vi "send&receive_2_arrs, call foo.vi"() -> ()   [LabVIEW 2018, in "LV2Julia_core.lvlib"]
uses:
  LV2Julia_core.lvlib
  Commands.ctl
  commands LV2Jl.ctl
  Server or client state.ctl
  d2cb43a9-9305-42fb-ad58-bce983510195.vi
  5398bb44-7854-4704-a5a4-70900ab1788b.vi
  4837e4b1-53a7-49b6-9aef-263877b89a45.vi
  464ea3ce-3b02-4d89-9aac-48d52021810b.vi
  edf81fa3-46bf-427f-9605-85b461656974.vi
  StackFrame.ctl
  detailed error info.ctl
panel:
  out "resp1":dbl
  in  "arg2":string
  in  "arg1":dbl
  in  "1D Array of I16":i16[](array[numeric])=[13, 7, 546]
  in  "2D Array of Cx32":csg[][](array[numeric])=[[3.0+0.0i, 1.0+1.0i], [0.0+7.0i, 1.0+4.0i]] format="%#_13g"
  out "resp2":i32[](array[numeric])
  in  "next":bool
  in  "stop LV only":bool
  in  "stop":bool
  out "detailed error info":T1
  out "resp3":dbl[](array[numeric])
  out "Jl Server state out":T3
  out "short err code":u8
  out "final error":errorcluster
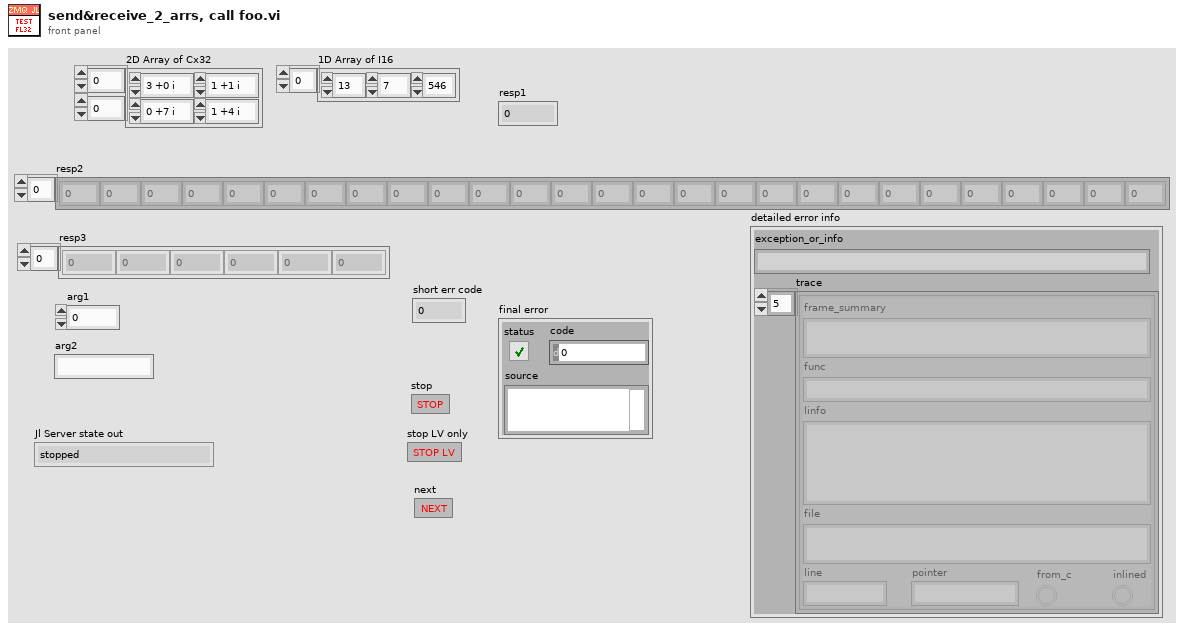
[diagram p1: front panel]
types:
  T1 = typedef "LV-0mq-Julia_roundtrip-lib.lvlib/detailed error info.ctl" = cluster{"exception_or_info":string, "trace":T2[]}
  T2 = typedef "LV-0mq-Julia_roundtrip-lib.lvlib/StackFrame.ctl" = cluster{"frame_summary":string, "func":string, "linfo":string, "file":string, "line":i32, "pointer":u64, "from_c":bool, "inlined":bool}
  T3 = typedef "LV-0mq-Julia_roundtrip-lib.lvlib/Server or client state.ctl" = enum16{"stopped", "running", "unknown"}
  T4 = typedef "LV-0mq-Julia_roundtrip-lib.lvlib/Commands.ctl" = enum16{"Start Jl-server & Init LV-client", "Send request & Get response ", "Stop Jl-server & Cleanup LV-client", "Cleanup LV-client", "Start Jl-server", "Stop Jl-server", "Init LV-Client", "Cleanup LV-Client", "(not allowed)", "Set LV Client state", "Set Jl Server state", "set ZMQ timeout", "read ZMQ timeout", "read-out state"}
  T5 = typedef "LV-0mq-Julia_roundtrip-lib.lvlib/commands LV2Jl.ctl" = u8
  T6 = typedef "LV-0mq-Julia_roundtrip-lib.lvlib/Bindata&description.ctl" = cluster{"bindata_descr":T7[], "bindata":u8[]}
  T7 = typedef "LV-0mq-Julia_roundtrip-lib.lvlib/Bindata description.ctl" = cluster{"nofbytes":i32, "numtype":string, "start":i32, "arrdims":i32[], "kwarg_name":string, "category":string}
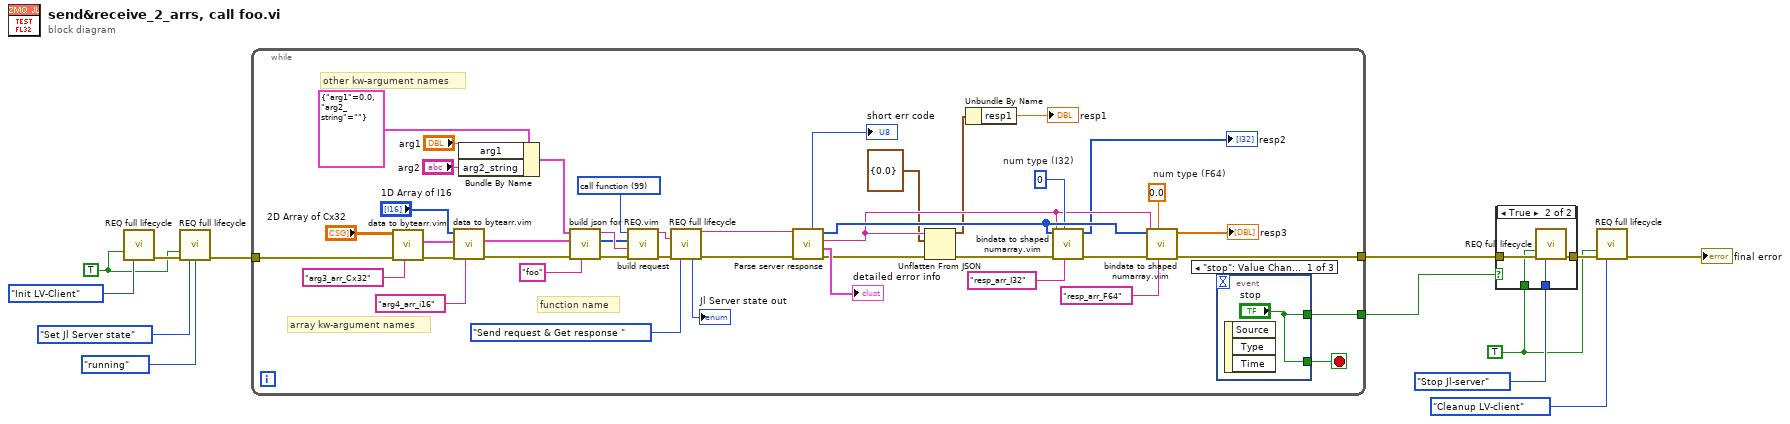
[diagram p0: block diagram]
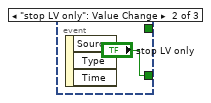
[diagram p2: hidden frame]
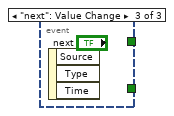
[diagram p3: hidden frame]
diagram:
  w4 = TRUE ("Force command")
  w8 = TRUE ("Force command")
  n1 = call "REQ full lifecycle.vi"("Force command"=w4, "command"=Commands."Init LV-Client") -> ("error out"=w6:errorcluster)  [unwired: 7 in, 6 out]
  n2 = call "REQ full lifecycle.vi"("Force command"=w4, "error in"=w6, "command"=Commands."Set Jl Server state", "Jl Server state in"=Server_or_client_state."running") -> ("error out"=w2:errorcluster)  [unwired: 5 in, 6 out]
  n3 = while {
    tunnel: w2 -> [w25]
    tunnel: [w41] -> w13
    tunnel: [w42] -> w1
    stop <- w43 stop-if-true
    w37 = 0  # num type (I32)
    w40 = 0.0  # num type (F64)
    w50 = T5 99 items=["call function"=99, "ping"=112, "stop"=115] ("Command")
    # "function name"
    # "other kw-argument names"
    # "array kw-argument names"
    n4 = call "data to bytearr.vim"("kwarg_name"="arg3_arr_Cx32", "error in (no error)"=w25, "data in"="2D Array of Cx32") -> ("error out"=w29:errorcluster, "Bindata & descr out"=w28:T6)  [unwired: 6 in, 1 out]
    n5 = call "data to bytearr.vim"("kwarg_name"="arg4_arr_i16", "error in (no error)"=w29, "Bindata & descr in"=w28, "data in"="1D Array of I16") -> ("error out"=w26:errorcluster, "Bindata & descr out"=w27:T6)  [unwired: 5 in, 1 out]
    n6 = Bundle By Name(cluster=cluster{"arg1":dbl, "arg2_string":string} {"arg1"=0.0, "arg2_string"=""}, "arg1"="arg1", "arg2_string"="arg2") -> (w21:cluster{"arg1":dbl, "arg2_string":string})
    n7 = call "build json for REQ.vim"("fun2call"="foo", "Bindata & descr in"=w27, "error in (no error)"=w26, "Arguments 1"=w21) -> ("error out"=w55:errorcluster, "bindata out"=w46:u8[], "JSON string out"=w47:string)  [unwired: 5 in]
    n8 = call "build request.vi"("error in (no error)"=w55, "JSON data"=w47, "binary data"=w46, "Command"=w50) -> ("error out"=w53:errorcluster, "REQ string"=w54:string)  [unwired: 6 in]
    n9 = call "REQ full lifecycle.vi"("data to send"=w54, "error in"=w53, "command"=Commands."Send request & Get response ") -> ("server response"=w14:string, "Jl Server state out"=→"Jl Server state out":T3, "error out"=w52:errorcluster)  [unwired: 6 in, 4 out]
    n10 = call "Parse server response.vi"("error in (no error)"=w52, "server response in"=w14) -> ("error out"=w44:errorcluster, "detailed error info"=→"detailed error info":T1, "JSON out"=w36:string, "binary data"=w39:u8[], "return code"=→"short err code":u8)  [unwired: 2 in, 3 out]
    n11 = Unflatten From JSON(JSON string=w36, type and defaults=cluster{"resp1":dbl} {"resp1"=0.0} ("parsed response"), error in (no error)=w44) -> (value=w31:cluster{"resp1":dbl}, error out=w33:errorcluster)  [unwired: 4 in]
    n12 = Unbundle By Name(w31) -> ("resp1"=→"resp1":dbl)
    n13 = call "bindata to shaped numarray.vim"("name"="resp_arr_I32" ("kwarg_name"), "data type"=w37, "error in (no error)"=w33, "binary data"=w36, "JSON in"=w39) -> ("error out"=w38:errorcluster, "numarray 1D"=→"resp2":i32[])  [unwired: 3 in, 2 out]
    n14 = call "bindata to shaped numarray.vim"("name"="resp_arr_F64" ("Tag"), "data type"=w40, "error in (no error)"=w38, "binary data"=w36, "JSON in"=w39) -> ("error out"=w41:errorcluster, "numarray 1D"=→"resp3":dbl[])  [unwired: 3 in, 2 out]
    n15 = event shown="[0] \"stop\": Value Change" {
      selector: _ -> [_ _ _]
      dyn-events: _ -> [_ _ _]
      timeout: _ -> [_ _ _]
      tunnel: ["stop" "stop LV only" _] -> w43
      tunnel: ["stop" _ _] -> w42
      event "stop": Value Change {
        n16 = event-data() -> ()  [unwired: 1 in, 3 out]
      }
      event "stop LV only": Value Change {
        n17 = event-data() -> ()  [unwired: 1 in, 3 out]
      }
      event "next": Value Change {
        n18 = event-data() -> ()  [unwired: 1 in, 3 out]
      }
    }
  }
  n19 = case shown="True" w1 {
    tunnel: w13 -> [w59 w63]
    tunnel: Commands."Stop Jl-server" ("command") -> [_ w62]
    tunnel: [w59 w61] -> w11
    tunnel: w8 -> [_ w60]
    frame False {
    }
    frame True {
      n20 = call "REQ full lifecycle.vi"("Force command"=w60, "error in"=w63, "command"=w62) -> ("error out"=w61:errorcluster)  [unwired: 6 in, 6 out]
    }
  }
  n21 = call "REQ full lifecycle.vi"("Force command"=w8, "error in"=w11, "command"=Commands."Cleanup LV-client") -> ("error out"=→"final error":errorcluster)  [unwired: 6 in, 6 out]
